vi "createrandom.vi"() -> (3 "Array":i32[][](array[numeric]))   [LabVIEW 2018]
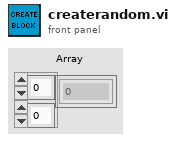
[diagram p1: front panel]
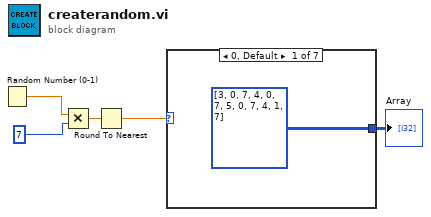
[diagram p0: block diagram]
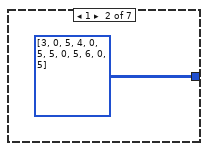
[diagram p2: hidden frame]
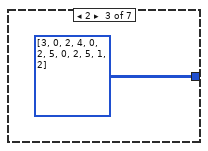
[diagram p3: hidden frame]
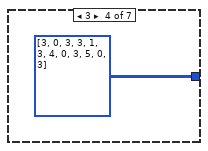
[diagram p4: hidden frame]
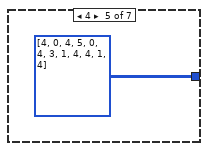
[diagram p5: hidden frame]
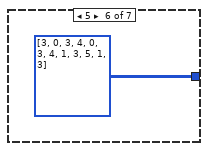
[diagram p6: hidden frame]
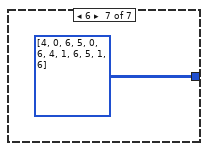
[diagram p7: hidden frame]
diagram:
  n1 = Random Number (0-1)() -> (number: 0 to 1=w5:dbl)
  n2 = Multiply(x=w5, y=7) -> (x*y=w3:dbl)
  n3 = Round To Nearest(number=w3) -> (nearest integer value=w2:dbl)
  n4 = case shown="0, Default" w2 {
    tunnel: [i32[][] [[3, 0, 7], [4, 0, 7], [5, 0, 7], [4, 1, 7]] i32[][] [[3, 0, 5], [4, 0, 5], [5, 0, 5], [6, 0, 5]] i32[][] [[3, 0, 2], [4, 0, 2], [5, 0, 2], [5, 1, 2]] i32[][] [[3, 0, 3], [3, 1, 3], [4, 0, 3], [5, 0, 3]] i32[][] [[4, 0, 4], [5, 0, 4], [3, 1, 4], [4, 1, 4]] i32[][] [[3, 0, 3], [4, 0, 3], [4, 1, 3], [5, 1, 3]] i32[][] [[4, 0, 6], [5, 0, 6], [4, 1, 6], [5, 1, 6]]] -> w1
    frame 0, Default {
    }
    frame 1 {
    }
    frame 2 {
    }
    frame 3 {
    }
    frame 4 {
    }
    frame 5 {
    }
    frame 6 {
    }
  }
  "Array" <- w1
